vi "Unregistration.vi"(10 "Registration":refnum<event-registration>) -> (2 "Remaining":refnum<class "Msg Strategy.lvclass">[](array[class]))   [LabVIEW 2021, in "jettl.lvlib" / "Self Event.lvlib"]
uses:
  Self Event.lvlib
  Msg Strategy/Msg Strategy.lvclass
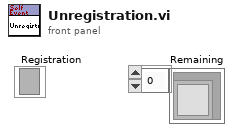
[diagram p1: front panel]
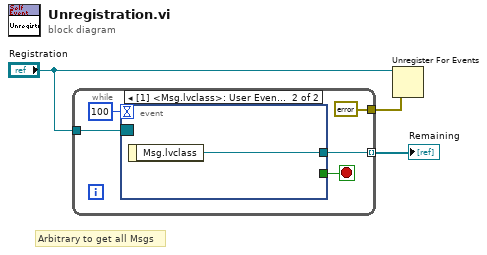
[diagram p0: block diagram]
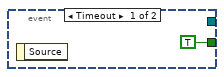
[diagram p2: hidden frame]
diagram:
  # "Arbitrary to get all Msgs"
  n1 = while {
    tunnel: "Registration" -> [w7]
    tunnel: [w5] -> w2 mode=indexing
    tunnel: [errorcluster {"status"=FALSE, "code"=0, "source"=""} ("error in (no error)")] -> w1
    stop <- w8 stop-if-true
    n2 = event shown="[1] <Msg.lvclass>: User Event" {
      selector: w7 -> [_ _]
      dyn-events: _ -> [_ _]
      timeout: 100 -> [_ _]
      tunnel: [TRUE _] -> w8
      tunnel: [_ w10] -> w5
      event Timeout {
        n3 = event-data() -> ()  [unwired: 1 in, 1 out]
      }
      event User Event {
        n4 = event-data() -> ("Msg.lvclass"=w10:refnum<class "Msg Strategy.lvclass">)  [unwired: 1 in]
      }
    }
  }
  "Remaining" <- w2
  n5 = Unregister For Events(event registration refnum="Registration", error in=w1) -> ()  [unwired: 1 out]
